vi "NLDBIFUR.VI"() -> ()   [LabVIEW 2012]
doc: "This program builds a bifurcation diagram of the driven PN-junction. For each value of the driving amplitude V, the current is sampled synchronously. There are two controls on the Jefferies box that will change what you see: the GAIN pot, and the STROBE PHASE CONTROLLER DELAY pot. The GAIN pot is in series with the driving oscillator, so make sure it's as high as it will go (all the way clock-wise). The DELAY pot controls where in the cycle of the drive oscillator the PN-junction is sampled. Varying it amount to slicing the attractor at different places. You can see this on the oscilloscope: the bright dots are where the ADC will sample the pn-junction current."
uses:
  <vilib>/DAQmx/write.llb/DAQmx Write (Analog DBL 1Chan 1Samp).vi
  <vilib>/DAQmx/miscellaneous.llb/DAQmx Fill In Error Info.vi
panel:
  out "Warning\nMessage":string="WARNING:  The increment in voltage along the horizontal axis is 2E+4 microV.  This is getting close (order of magnitude) to the limitation  (153 microV) of the data-acquisition card."
  in  "Conversion Trigger Source":enum16{"Internal", "External"}(ring)=enum."External"
  out "Progress":dbl(slide)=4.298736016932021 scale=0.0..10.0 scale format="%.2f"
  in  "# of points":i16=250
  out "System response as a function of driving voltage":cluster{sgl, sgl}[](graph)
  in  "V Stop":dbl=4.316000017 step=0.01 format="%.8f"
  in  "V Start":dbl step=0.01 format="%.8f"
  in  "Number of points per value of V":i16=100 step=50
  # "Bifurcation Diagram"
  # "Select 'Get Info' from the 'file' menu for more about this program"
  # "Press the run button and turn off the monitor for best stability."
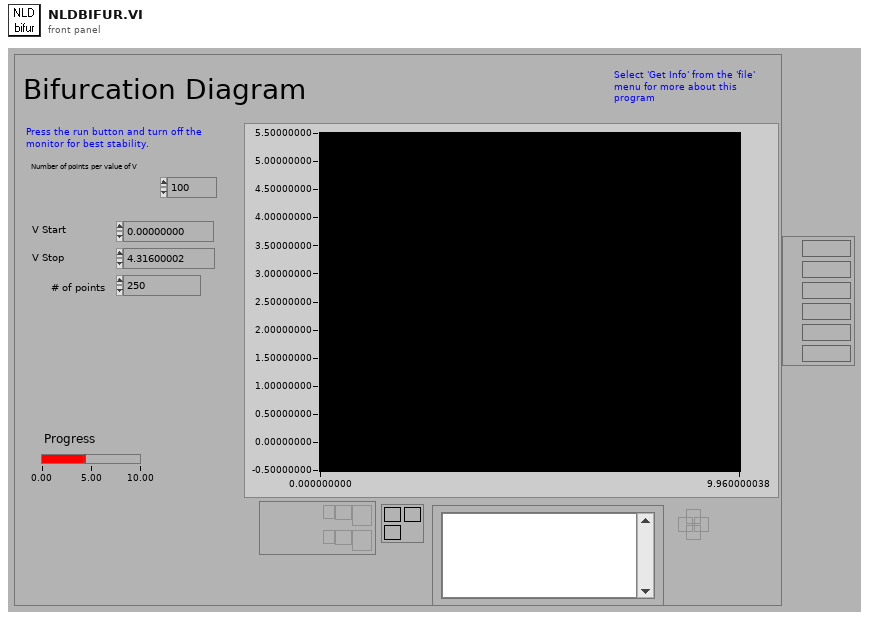
[diagram p1: front panel]
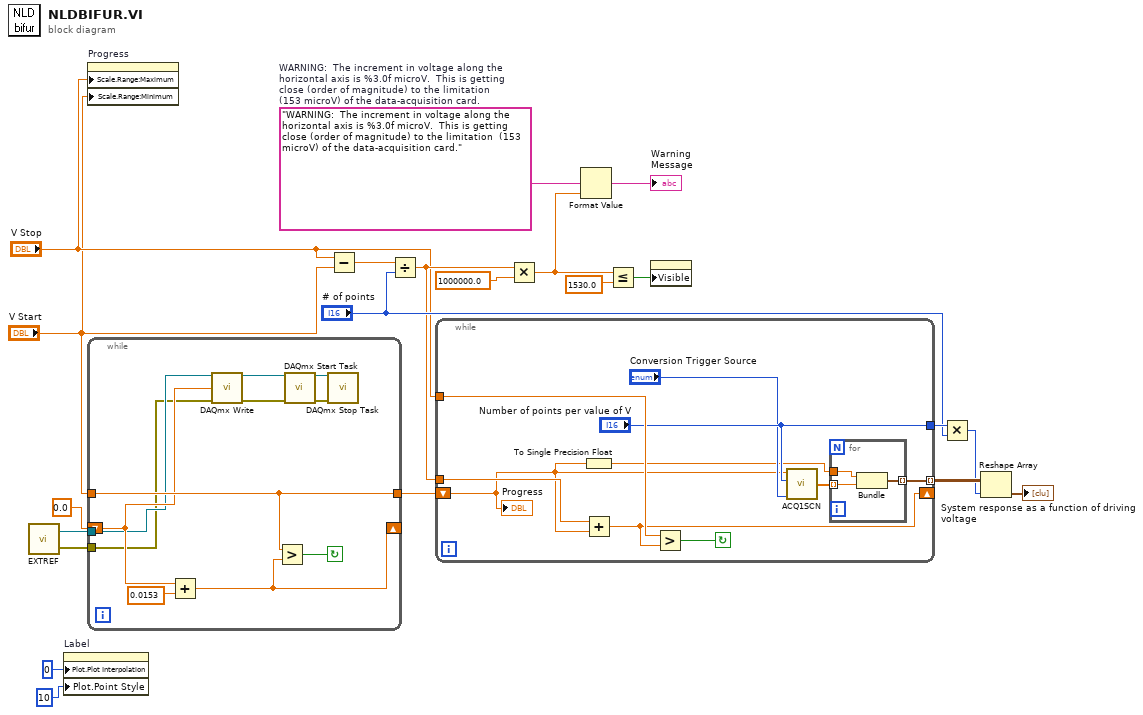
[diagram p0: block diagram]
diagram:
  w12 = "WARNING:  The increment in voltage along the horizontal axis is %3.0f microV.  This is getting close (order of magnitude) to the limitation  (153 microV) of the data-acquisition card."  # WARNING:  The increment in voltage along the horizontal axis is %3.0f microV.  This is getting close (order of magnitude) to the limitation  (153 microV) of the data-acquisition card.
  n1 = call "EXTREF.vi"() -> ("error out"=w3:errorcluster, "task out"=w4:refnum<k21>)  [unwired: 2 in]
  n2 = property on="Label" class="XYGraph (strict)"("Plot.Plot Interpolation"=0, "Plot.Point Style"=10) -> ()  [unwired: 2 in, 2 out]
  n3 = property on="Progress" class="Slide (strict)"("Scale.Range:Maximum"="V Stop", "Scale.Range:Minimum"="V Start") -> ()  [unwired: 2 in, 2 out]
  n4 = while {
    tunnel: [w29] -> w5
    tunnel: "V Start" -> [w29]
    shift-left: 0.0 -> [w24]
    shift-right: [w30] -> _
    tunnel: w4 -> [w23]
    tunnel: w3 -> [w22]
    stop <- w31 continue-if-true
    n5 = Add(x=w24, y=0.0153) -> (x+y=w30:dbl)
    n6 = call-poly <vilib>:"DAQmx Write.vi"("task/channels in"=w23, "data"=w24, "error in"=w22) -> ("task out"=w28:refnum<k21>, "error out"=w27:errorcluster)  [unwired: 10 in, 1 out]
    n7 = Greater?(x=w29, y=w30) -> (0:w31:bool)
    n8 = call <vilib>:"DAQmx Start Task.vi"("task/channels in"=w28, "error in"=w27) -> ("task out"=w25:refnum<k21>, "error out"=w26:errorcluster)  [unwired: 12 in]
    n9 = call <vilib>:"DAQmx Stop Task.vi"("task/channels in"=w25, "error in"=w26) -> ()  [unwired: 12 in, 2 out]
  }
  n10 = Subtract(x="V Stop", y="V Start") -> (x-y=w18:dbl)
  n11 = Divide(x=w18, y="# of points") -> (x/y=w13:dbl)
  n12 = while {
    tunnel: ["Number of points per value of V"] -> w17
    tunnel: "V Stop" -> [w38]
    tunnel: w13 -> [w39]
    tunnel: [w40] -> w19 mode=indexing
    shift-left: w5 -> [w34]
    shift-right: [w37] -> _
    stop <- w42 continue-if-true
    n13 = To Single Precision Float(number=w34) -> (single precision float=w33:sgl)
    n14 = Add(x=w39, y=w34) -> (x+y=w37:dbl)
    n15 = Greater?(x=w38, y=w37) -> (0:w42:bool)
    n16 = call "ACQ1SCN.VI"("Conversion Trigger Source"="Conversion Trigger Source", "buffer size"="Number of points per value of V", "Chaotic Param (R)"=w34) -> ("Sampled Data"=w41:sgl[])  [unwired: 1 in]
    n17 = for {
      tunnel: w41 -> [w44] mode=indexing
      tunnel: [w45] -> w40 mode=indexing
      tunnel: w33 -> [w43]
      n18 = Bundle(w43, w44) -> (w45:cluster{sgl, sgl})  [unwired: 1 in]
    }
    "Progress" <- w34
  }
  n19 = Multiply(x=w13, y=1000000.0) -> (x*y=w9:dbl)
  n20 = Format Value(format string=w12, value (0)=w9) -> (output string=→"Warning\nMessage":string)  [unwired: 1 in]
  n21 = Less Or Equal?(x=w9, y=1530.0) -> (x <= y?=w7:bool)
  n22 = property on="Warning\nMessage" class="Str"("Visible"=w7) -> ()  [unwired: 2 in, 2 out]
  n23 = Multiply(x=w17, y="# of points") -> (x*y=w16:i16)
  n24 = Reshape Array(w19, w16) -> (→"System response as a function of driving voltage":cluster{sgl, sgl}[])
